vi "Send Configure FM Internal [FM].vi"(6 "modulation waveform (Sine)":i32(ring)=1 items=["Sine"=1, "Square"=2, "Triangle"=3, "Ramp Up"=4, "Ramp Down"=5], 7 "Message Priority (Normal)":T1=enum."Normal", 8 "error in (no error)":errorcluster, 9 "modulation frequency (1000 Hz)":dbl[unit]=1000.0 format="%^.2e", 10 "peak deviation (100 Hz)":dbl[unit]=100.0 format="%^.2e", 11 "Message Enqueuer":refnum<class "Message Enqueuer.lvclass">) -> (0 "error out":errorcluster, 3 "Message Enqueuer out":refnum<class "Message Enqueuer.lvclass">)   [LabVIEW 2015, in "CS++Fgen.lvlib" / "Configure FM Internal [FM] Msg.lvclass"]
doc: "Sends the <B>CS++Fgen.lvlib:Configure FM Internal [FM] Msg.lvclass</B> message.\n\n<B>CS++Fgen.lvlib:CS++Fgen.lvclass:Configure FM Internal [FM].vi</B> Description:\n\nThis VI configures the properties that control the function generator's internal frequency modulation source. These properties are the peak deviation, waveform, and frequency.\n\nNotes:\n\n(1) This VI is part of the IviFgenModulateFM [FM] extension group."
uses:
  Configure FM Internal [FM] Msg.lvclass
  <vilib>/ActorFramework/Message Enqueuer/Message Enqueuer.lvclass
  <vilib>/ActorFramework/Message Enqueuer/Message Priority.ctl
  Configure FM Internal [FM] Msg.lvclass/Configure FM Internal [FM] Msg.ctl
  <vilib>/ActorFramework/Message Enqueuer/Message Enqueuer.lvclass/Message Enqueuer.ctl
  <vilib>/ActorFramework/Message Priority Queue/Priority Enqueue.vi
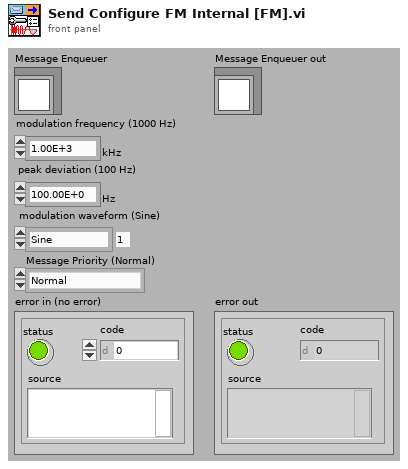
[diagram p1: front panel]
types:
  T1 = typedef "Actor Framework.lvlib/Message Enqueuer.lvclass/Message Priority.ctl" = enum16{"Low", "Normal", "High"}
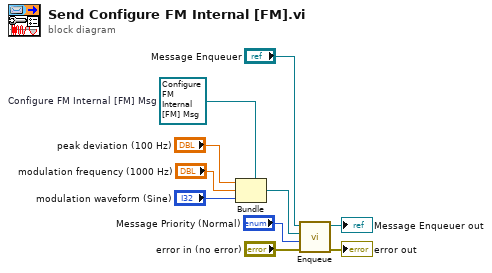
[diagram p0: block diagram]
diagram:
  w4 = refnum<class "Configure FM Internal [FM] Msg.lvclass"> refnum  # Configure FM Internal [FM] Msg
  n1 = Bundle(cluster=w4, "peak deviation (100 Hz)", "modulation frequency (1000 Hz)", "modulation waveform (Sine)") -> (w7:refnum<class "Configure FM Internal [FM] Msg.lvclass">)
  n2 = call <vilib>:"Enqueue.vi"("error in (no error)"="error in (no error)", "Message Priority (Normal)"="Message Priority (Normal)", "Message"=w7, "Message Enqueuer in"="Message Enqueuer") -> ("error out"=→"error out":errorcluster, "Message Enqueuer out"=→"Message Enqueuer out":refnum<class "Message Enqueuer.lvclass">)  [unwired: 6 in]
